vi "writeToXML.vi"(8 "error in (no error)":errorcluster, 10 "ClassLabel":string, 11 "RotOffset in":refnum<class "RotOffset.lvclass">) -> (0 "error out":errorcluster, 2 "XML out":string, 3 "RotOffset out":refnum<class "RotOffset.lvclass">)   [LabVIEW 2022 SP3, in "TCSDataDefinitions.lvlib" / "TCSCommand.lvlib" / "OffsetCommands.lvlib" / "RotOffset.lvclass"]
uses:
  RotOffset.lvclass
  RotOffset.lvclass/RotOffset.ctl
  RotatorOffsetCommands/RotatorOffsetCommands.lvclass
  <userlib>/Common/XML/XMLGenerator/XMLGenerator.lvclass
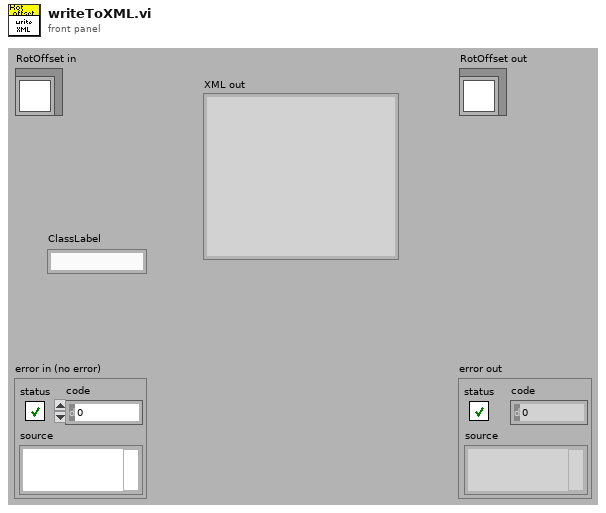
[diagram p1: front panel]
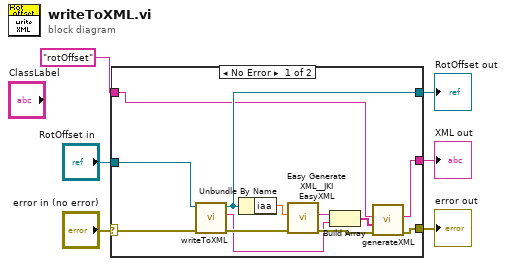
[diagram p0: block diagram]
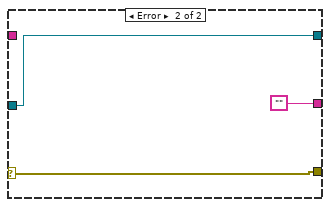
[diagram p2: hidden frame]
diagram:
  n1 = case shown="No Error" "error in (no error)" {
    selector: "error in (no error)" -> [w17 w21]
    tunnel: [w10 w21] -> w5
    tunnel: [w16 w20] -> w3
    tunnel: "RotOffset in" -> [w18 w20]
    tunnel: [w9 ""] -> w2
    tunnel: "rotOffset" ("ClassLabel") -> [w8 _]
    frame No Error {
      n2 = call-parent "writeToXML.vi"("error in (no error)"=w17, "RotatorOffsetCommands in"=w18) -> ("error out"=w14:errorcluster, "XML out"=w7:string, "RotatorOffsetCommands out"=w16:refnum<class "RotOffset.lvclass">)  [unwired: 7 in]
      n3 = Unbundle By Name(w16) -> ("iaa"=w15:dbl[unit])
      n4 = call <vilib>:"Easy Generate XML__JKI EasyXML.vi"("error in (no error)"=w14, "LabVIEW Data"=w15) -> ("error out"=w11:errorcluster, "XML String"=w13:string)  [unwired: 8 in]
      n5 = Build Array(w13, w7) -> (w12:string[])
      n6 = call <userlib>:"generateXML.vi"("error in"=w11, "childrenXML"=w12, "elementName"=w8) -> ("error out"=w10:errorcluster, "XML out"=w9:string)  [unwired: 6 in, 1 out]
    }
    frame Error {
    }
  }
  "error out" <- w5
  "RotOffset out" <- w3
  "XML out" <- w2
